vi "Refresh IRQ Listbox.vi"(8 "IRQ Settings Array":T1[](array[typedef]), 11 "IRQ Listbox Refnum":refnum<vi>) -> ()   [LabVIEW 2016]
uses:
  <vilib>/Powertrain Controls/Device Drivers/DCM/IRQ/RT/IRQ Setup.ctl
  <vilib>/Powertrain Controls/Device Drivers/DCM/IRQ/RT/DCM - RT - IRQ.lvlib
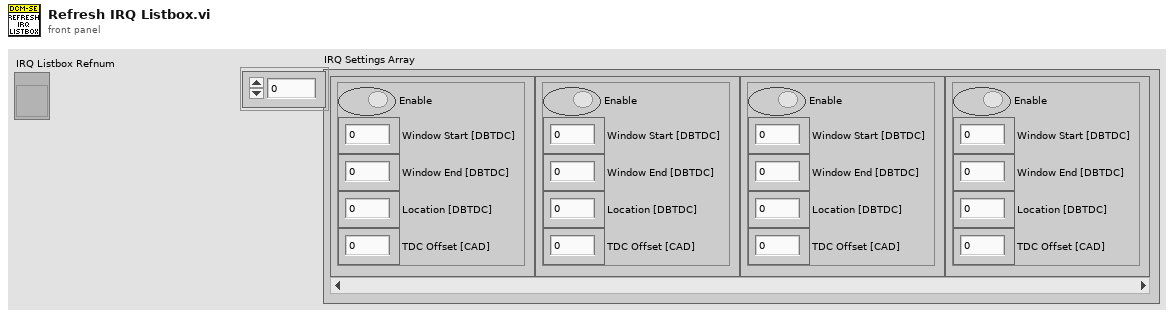
[diagram p1: front panel]
types:
  T1 = typedef "DCM - RT - IRQ.lvlib/IRQ Setup.ctl" = cluster{"Enable":bool, "Window Start [DBTDC]":sgl, "Window End [DBTDC]":sgl, "Location [DBTDC]":sgl, "TDC Offset [CAD]":sgl}
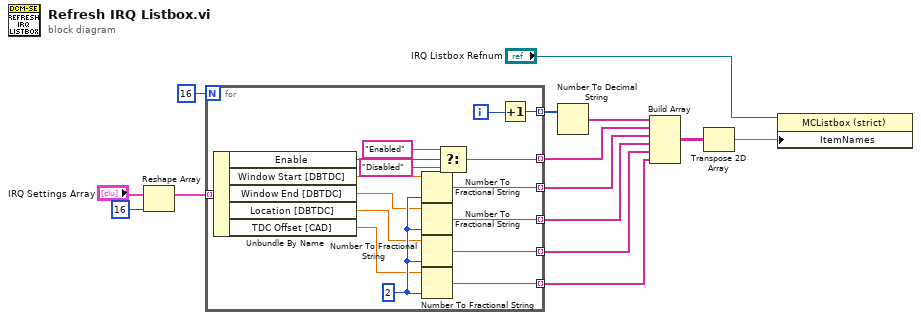
[diagram p0: block diagram]
diagram:
  n1 = Reshape Array("IRQ Settings Array", 16) -> (w12:T1[])
  n2 = for {
    N: 16 -> [_]
    tunnel: w12 -> [w28] mode=indexing
    tunnel: [w30] -> w9 mode=indexing
    tunnel: [w24] -> w5 mode=indexing
    tunnel: [w22] -> w4 mode=indexing
    tunnel: [w17] -> w3 mode=indexing
    tunnel: [w16] -> w2 mode=indexing
    tunnel: [w15] -> w1 mode=indexing
    i -> [w29]
    w21 = i16 2 ("precision (6)")
    n3 = Unbundle By Name(w28) -> ("Enable"=w27:bool, "Window Start [DBTDC]"=w23:sgl, "Window End [DBTDC]"=w20:sgl, "Location [DBTDC]"=w19:sgl, "TDC Offset [CAD]"=w18:sgl)
    n4 = Number To Fractional String(number=w23, precision (6)=w21) -> (F-format string=w22:string)  [unwired: 2 in]
    n5 = Number To Fractional String(number=w20, precision (6)=w21) -> (F-format string=w17:string)  [unwired: 2 in]
    n6 = Number To Fractional String(number=w19, precision (6)=w21) -> (F-format string=w16:string)  [unwired: 2 in]
    n7 = Number To Fractional String(number=w18, precision (6)=w21) -> (F-format string=w15:string)  [unwired: 2 in]
    n8 = Select(t="Enabled", s=w27, f="Disabled") -> (s? t:f=w24:string)
    n9 = Increment(x=w29) -> (x+1=w30:i32)
  }
  n10 = Number To Decimal String(number=w9) -> (decimal integer string=w10:string[])  [unwired: 1 in]
  n11 = Build Array(w10, w5, w4, w3, w2, w1) -> (w14:string[][])
  n12 = Transpose 2D Array(2D array=w14) -> (transposed array=w8:string[][])
  n13 = property on="Property Node" class="MCListbox (strict)"(reference="IRQ Listbox Refnum", "ItemNames"=w8) -> ()  [unwired: 1 in, 2 out]
